vi "Launch View.vi"(8 "error in (no error)":errorcluster, 9 "Timeout [ms] (-1)":i32=-1, 11 "View In":refnum<class "View.lvclass">) -> (0 "error out":errorcluster, 1 "Timed out?":bool, 3 "View Out":refnum<class "View.lvclass">)   [LabVIEW 2020, in "View.lvclass"]
uses:
  View.lvclass
  C:/git/astemes-triarc-framework/source/Framework/Process/Process.lvclass
  View.lvclass/View.ctl
  Process/Process.lvclass
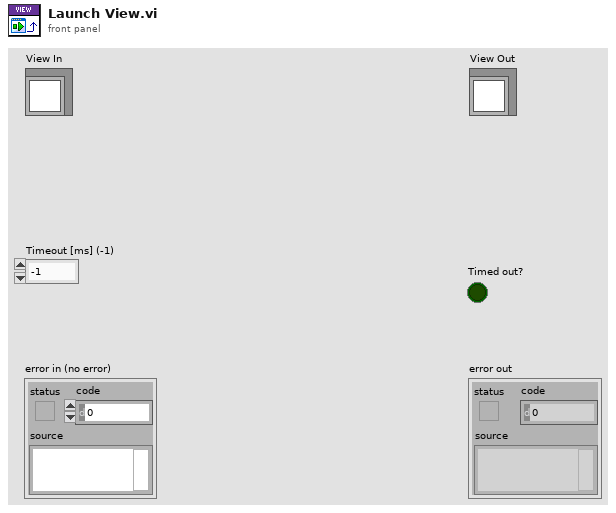
[diagram p1: front panel]
types:
  T1 = typedef "Process.lvclass/Lifecycle State.ctl" = enum16{"Uninitialized", "Initialized", "Started", "Running", "Stopped", "Finished"}
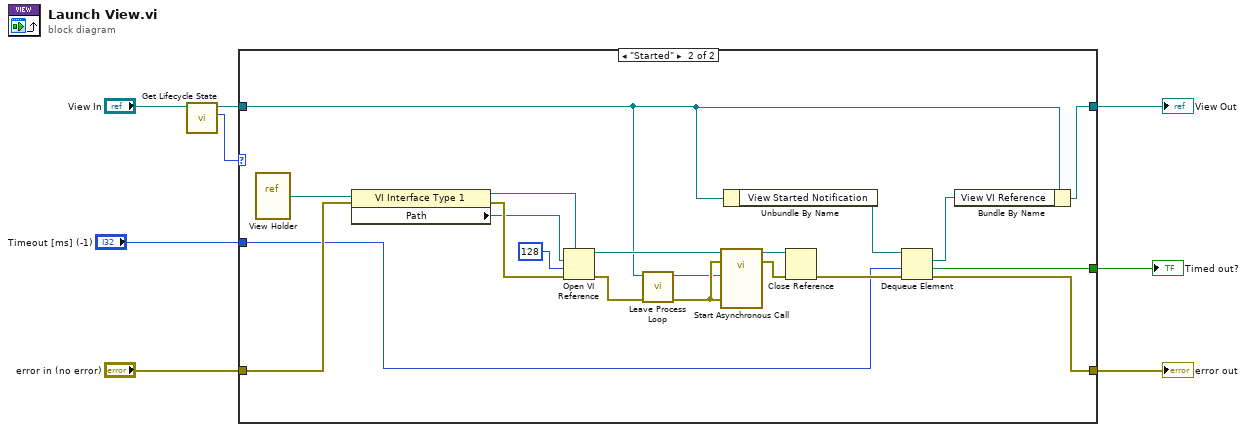
[diagram p0: block diagram]
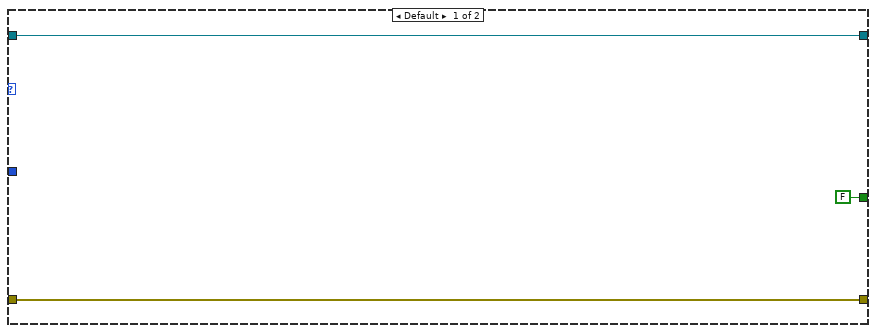
[diagram p2: hidden frame]
diagram:
  n1 = call "Get Lifecycle State.vi"("Process In"="View In") -> ("Lifecycle State"=w1:T1, "Process Out"=w2:refnum<class "View.lvclass">)  [unwired: 7 in, 2 out]
  n2 = case shown="\"Started\"" w1 {
    tunnel: "error in (no error)" -> [w9 w27]
    tunnel: [w9 w22] -> w7
    tunnel: [w11 w20] -> w6
    tunnel: [FALSE ("timed out?") w19] -> w5
    tunnel: "Timeout [ms] (-1)" -> [_ w17]
    tunnel: w2 -> [w11 w12]
    frame Default {
    }
    frame "Started" {
      n3 = vi-ref "View Holder.vi"() -> (w13:refnum<vi>)
      n4 = property class="VI Interface Type 1"(reference=w13, error in=w27) -> (reference out=w25:refnum<vi>, error out=w31:errorcluster, "Path"=w28:path)
      n5 = Open VI Reference(type specifier VI Refnum (for type only)=w25, vi path=w28, options=128, error in (no error)=w31) -> (vi reference=w30:refnum<vi>, error out=w16:errorcluster)  [unwired: 2 in]
      n6 = call "Leave Process Loop.vi"("error in (no error)"=w16, "Process In"=w12) -> ("error out"=w15:errorcluster, "Process Out"=w14:refnum<class "View.lvclass">)  [unwired: 8 in]
      n7 = call-by-ref "Start Asynchronous Call"(reference=w30, error in=w15, 8:"error in (no error)"=w15, "View in"=w14) -> (reference out=w24:refnum<vi>, error out=w26:errorcluster)  [unwired: 9 in, 1 out]
      n8 = Unbundle By Name(w12) -> ("View Started Notification"=w21:refnum<queue>)
      n9 = Close Reference(reference=w24, error in (no error)=w26) -> (error out=w23:errorcluster)
      n10 = Dequeue Element(queue=w21, timeout in ms (-1)=w17, error in (no error)=w23) -> (element=w18:refnum<vi>, timed out?=w19:bool, error out=w22:errorcluster)  [unwired: 1 out]
      n11 = Bundle By Name(cluster=w12, "View VI Reference"=w18) -> (w20:refnum<class "View.lvclass">)
    }
  }
  "error out" <- w7
  "View Out" <- w6
  "Timed out?" <- w5
